vi "LIN frame Generator for Test.vi"() -> ()   [LabVIEW 2025]
uses:
  <vilib>/xnet/xnet.llb/XNET Frame Type LIN.ctl
  <vilib>/xnet/xnet.llb/XNET Create Session (Frame Output Stream).vi
  <vilib>/xnet/xnet.llb/XNET Write (Frame LIN).vi
  <resource>/objmgr/xnet.rc
panel:
  in  "LIN frame":T2(array[cluster])=[{"timestamp"=timestamp(0 s since 1904-01-01), "payload"=[1, 2, 3, 4, 5], "identifier"=16, "type"=64, "event ID"=0, "event slot?"=FALSE, "echo?"=FALSE}] {"event ID" format="%x"; "payload" format="%x"; "timestamp" format="%<%.7X\n%x>T"; "type" items=["LIN Data"=64, "LIN Bus Error"=65, "LIN No Response"=66, "Delay"=224, "Log Trigger"=225, "Start Trigger"=226]; "identifier" format="%x"}
  in  "Wait time (ms)":u32=1000
  in  "Is Master Node":bool=TRUE
  in  "Baud Rate (bps)":u64=19200
  in  "Termination":bool
  in  "LIN interface":refnum<k21>
  out "Instruction":string="Sends LIN messages to the selected interface with the selected rate (defualt is 1000 ms).\nSet \"Is Master Node\" to true when no other master node active on the bus.\n"
  in  "Stop Button":bool
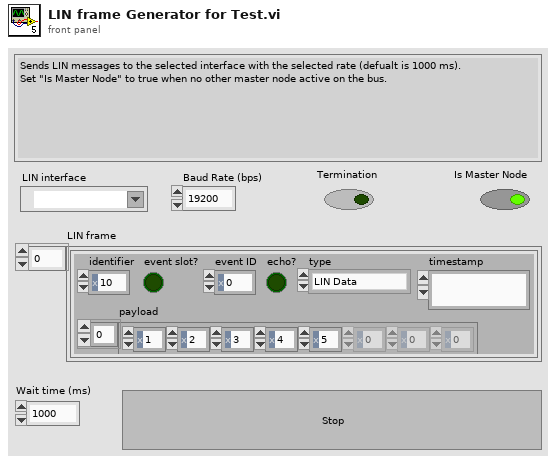
[diagram p1: front panel]
types:
  T1 = typedef "XNET Frame Type LIN.ctl" = u8
  T2 = cluster{"timestamp":timestamp, "payload":u8[], "identifier":u32, "type":T1, "event ID":u8, "event slot?":bool, "echo?":bool}[]
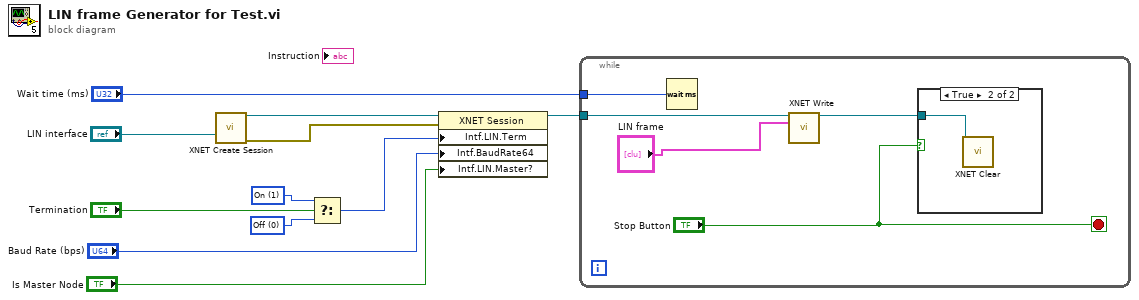
[diagram p0: block diagram]
diagram:
  w10 = u32 1 items=["Off", "On"] ("Interface:CAN:Termination")
  w11 = u32 0 items=["Off", "On"] ("Interface:CAN:Termination")
  n1 = call-poly <vilib>:"XNET Create Session.vi"("interface"="LIN interface") -> ("session out"=w7:refnum<k21>, "error out"=w8:errorcluster)  [unwired: 13 in]
  n2 = Select(t=w10, s="Termination", f=w11) -> (s? t:f=w9:u32)
  n3 = property class="XNET Session"(reference=w7, error in=w8, "Intf.LIN.Term"=w9, "Intf.BaudRate64"="Baud Rate (bps)", "Intf.LIN.Master?"="Is Master Node") -> (reference out=w2:refnum<k21>)  [unwired: 1 out]
  n4 = while {
    tunnel: w2 -> [w16]
    tunnel: "Wait time (ms)" -> [w13]
    stop <- "Stop Button" stop-if-true
    n5 = Wait (ms)(milliseconds to wait=w13) -> ()  [unwired: 1 out]
    n6 = call-poly <vilib>:"XNET Write.vi"("session in"=w16, "data"="LIN frame") -> ("session out"=w14:refnum<k21>)  [unwired: 12 in, 1 out]
    n7 = case shown="True" "Stop Button" {
      tunnel: w14 -> [_ w17]
      frame False {
      }
      frame True {
        n8 = call <vilib>:"XNET Clear.vi"("session in"=w17) -> ()  [unwired: 14 in, 1 out]
      }
    }
  }
